vi "Get Last PString.vi"(0 "String":string) -> (1 "Last String":string, 2 "PString Offset":i32)   [LabVIEW 2012, in "TD Tools.lvlib"]
uses:
  TD Tools.lvlib
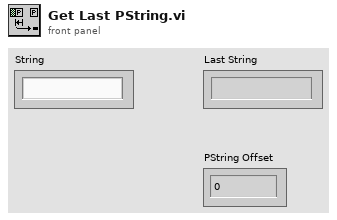
[diagram p1: front panel]
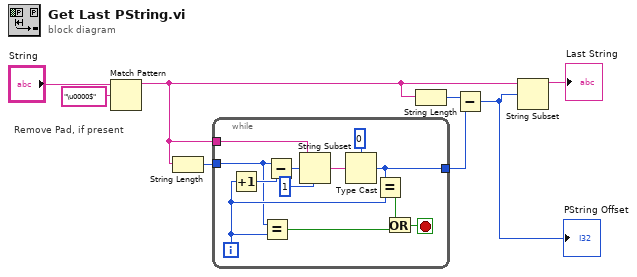
[diagram p0: block diagram]
diagram:
  # "Remove Pad, if present"
  n1 = Match Pattern(string="String", regular expression="\u0000$" ("*(type *) &x")) -> (before substring=w5:string)  [unwired: 1 in, 3 out]
  n2 = String Length(string=w5) -> (length=w4:i32)
  n3 = while {
    tunnel: [w15] -> w8
    tunnel: w4 -> [w10]
    tunnel: w5 -> [w19]
    i -> [w13]
    stop <- w12 stop-if-true
    n4 = Increment(x=w13) -> (x+1=w14:i32)
    n5 = Equal?(x=w10, y=w13) -> (x = y?=w9:bool)
    n6 = Subtract(x=w10, y=w14) -> (x-y=w18:i32)
    n7 = String Subset(string=w19, offset (0)=w18, length (rest)=1 ("length (rest)")) -> (substring=w17:string)
    n8 = Type Cast(type=u8 0, x=w17) -> (*(type *) &x=w15:u8)
    n9 = Equal?(x=w15, y=w13) -> (x = y?=w11:bool)
    n10 = Or(x=w11, y=w9) -> (x .or. y?=w12:bool)
  }
  n11 = String Length(string=w5) -> (length=w7:i32)
  n12 = Subtract(x=w7, y=w8) -> (x-y=w2:i32)
  "PString Offset" <- w2
  n13 = String Subset(string=w5, offset (0)=w2) -> (substring=→"Last String":string)  [unwired: 1 in]
